vi "Build between unit test strings.vi"(11 "all rows":string[](array[string])) -> (1 "Chaîne":string, 2 "Numérique":i32, 3 "Chaîne 2":string, 4 "Chaîne 4":string, 5 "Chaîne 3":string, 6 "Booléen":bool)   [LabVIEW 2021]
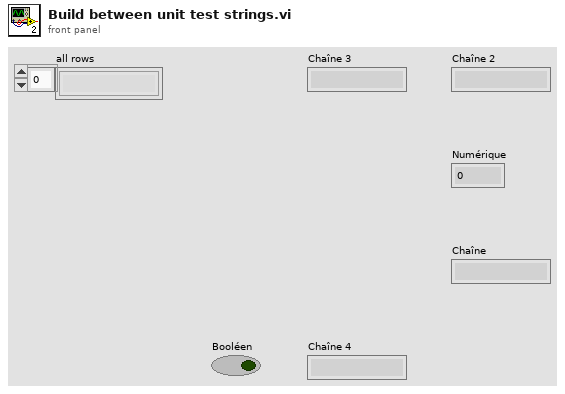
[diagram p1: front panel]
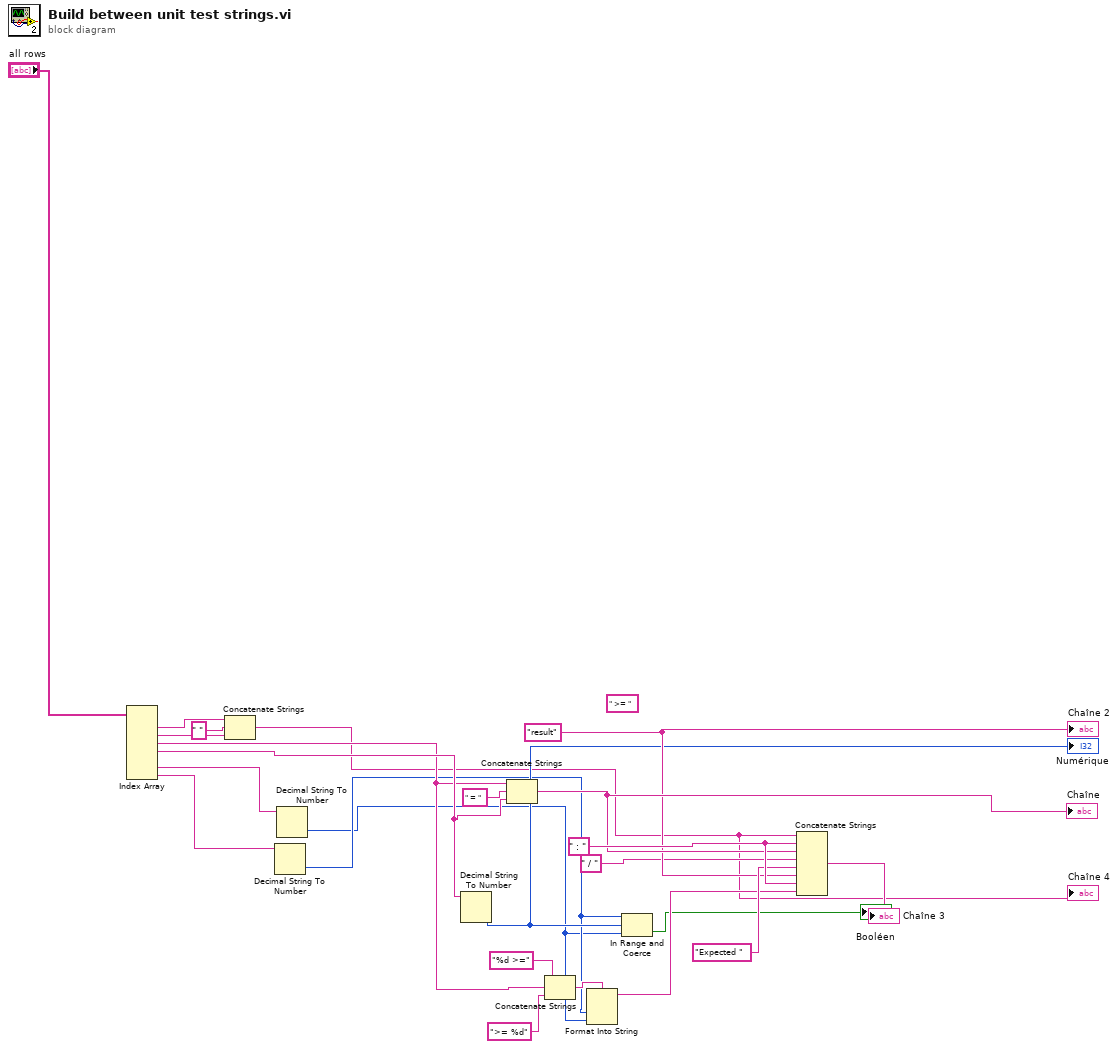
[diagram p0: block diagram]
diagram:
  w24 = " : " ("chaîne")
  (unwired) " >= " ("chaîne")
  w16 = "result"
  n1 = Index Array ("Indexer un tableau")(array="all rows") -> (element #1=w5:string, element #2=w3:string, element #3=w10:string, element #4=w11:string, element #6=w2:string, element #7=w6:string)  [unwired: 7 in, 1 out]
  n2 = Concatenate Strings ("Concaténer des chaînes")(w5, " " ("chaîne"), w3) -> (w7:string)
  "Chaîne 4" <- w7
  n3 = Decimal String To Number ("Chaîne décimale en nombre")(string=w6) -> (number=w9:i32)  [unwired: 2 in, 1 out]
  n4 = Decimal String To Number ("Chaîne décimale en nombre")(string=w2) -> (number=w8:i32)  [unwired: 2 in, 1 out]
  n5 = Decimal String To Number(string=w11) -> (number=w13:i32)  [unwired: 2 in, 1 out]
  "Numérique" <- w13
  n6 = Concatenate Strings(w10, " = " ("chaîne"), w11) -> (w22:string)
  "Chaîne" <- w22
  n7 = Concatenate Strings("%d >=" ("chaîne"), w10, ">= %d" ("chaîne")) -> (w17:string)
  n8 = Format Into String(format string=w17, w9, w8) -> (resulting string=w20:string)  [unwired: 2 in, 1 out]
  n9 = In Range and Coerce(upper limit=w9, x=w13, lower limit=w8) -> (In Range?=→"Booléen":bool)  [unwired: 1 out]
  n10 = Concatenate Strings(w7, w24, w22, " / " ("chaîne"), "Expected " ("chaîne"), w16, w24, w20) -> (→"Chaîne 3":string)
  "Chaîne 2" <- w16
